vi "Distance.vi"(1 "B":dbl[](array[numeric]), 2 "A":dbl[](array[numeric])) -> (0 "Distance":dbl)   [LabVIEW 2016]
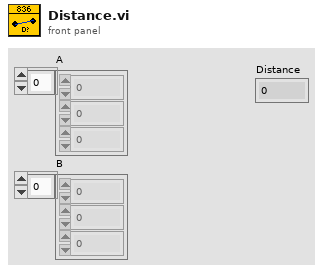
[diagram p1: front panel]
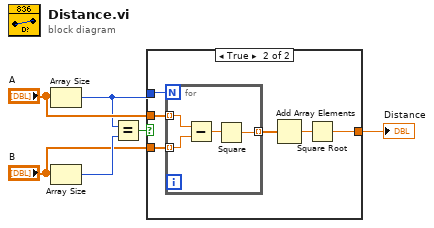
[diagram p0: block diagram]
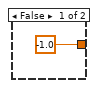
[diagram p2: hidden frame]
diagram:
  n1 = Array Size(array="A") -> (size(s)=w1:i32)
  n2 = Array Size(array="B") -> (size(s)=w6:i32)
  n3 = Equal?(x=w1, y=w6) -> (x = y?=w5:bool)
  n4 = case shown="True" w5 {
    tunnel: [-1.0 w8] -> w4
    tunnel: "A" -> [_ w13]
    tunnel: "B" -> [_ w12]
    tunnel: w1 -> [_ w11]
    frame False {
    }
    frame True {
      n5 = for {
        N: w11 -> [_]
        tunnel: w13 -> [w17] mode=indexing
        tunnel: w12 -> [w16] mode=indexing
        tunnel: [w14] -> w10 mode=indexing
        n6 = Subtract(x=w17, y=w16) -> (x-y=w15:dbl)
        n7 = Square(x=w15) -> (x^2=w14:dbl)
      }
      n8 = Add Array Elements(numeric array=w10) -> (sum=w9:dbl)
      n9 = Square Root(x=w9) -> (sqrt(x)=w8:dbl)
    }
  }
  "Distance" <- w4
